vi "Signal Recovery Lockin.vi"(1 "Action":T3=enum."Identify", 2 "Parameters":variant) -> (6 "Output":variant, 7 "Stop":bool)   [LabVIEW 2019]
uses:
  Sub Controls/Instrument Actions.ctl
  Sub Controls/Public.ctl
  Sub Controls/Instrument Match.ctl
  Sub Controls/Scan Output.ctl
  Sub Controls/Instrument IDN.ctl
  Sub Controls/User Event Command.ctl
  <vilib>/Instr/_visa.llb/VISA GPIB Control REN Mode.ctl
panel:
  in  "X/Y":bool=TRUE
  out "Title":string="Signal Recovery Lockin"
  in  "VISA resource name":refnum<visa-resource-name>
  in  "Instruments":T1[](array[typedef])=[{"Model"="7265", "Manufacturer"="Signal Recovery", "Term Character"="", "Wait Time (mS)"=0, "Wait for SRQ"=FALSE, "Type"="Lockin"}]
  out "Model":string
  in  "Address":u16(ring)
  in  "Channel":bool
  in  "Public":T2
  out "Measurement":dbl[](array[numeric]) format="%^.3e"
  # "Ch. 1&2"
  # "Ch. 1"
  # "Mag/Phase"
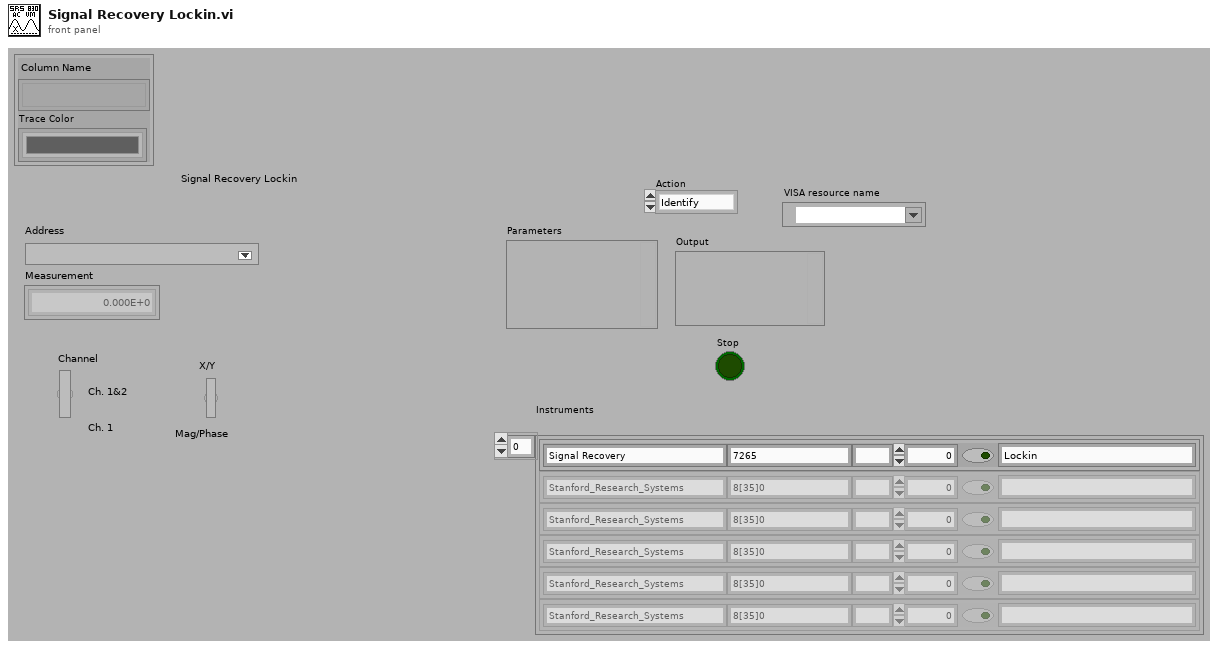
[diagram p1: front panel]
types:
  T1 = typedef "Instrument Match.ctl" = cluster{"Model":string, "Manufacturer":string, "Term Character":string, "Wait Time (mS)":u32, "Wait for SRQ":bool, "Type":string}
  T2 = typedef "Public.ctl" = cluster{"Column Name":string[], "Trace Color":u32[]}
  T3 = typedef "Instrument Actions.ctl" = enum16{"Scan", "Identify", "New", "Configure", "Initialize", "Test", "Read", "Close"}
  T4 = typedef "Scan Output.ctl" = cluster{"Manufacturer":string, "Model":string, "Info":string, "Revision":string, "error out":errorcluster}
  T5 = typedef "Instrument IDN.ctl" = cluster{"VISA Address":string, "Status":u16, "Manufacturer":string, "Model":string, "Info":string, "Info 2":string, "Misc Data":variant}
  T6 = typedef "User Event Command.ctl" = enum32{"Stop Config"}
  T7 = cluster{"VISA resource name":refnum<visa-resource-name>, string}
  T8 = typedef "VISA GPIB Control REN Mode.ctl" = u16
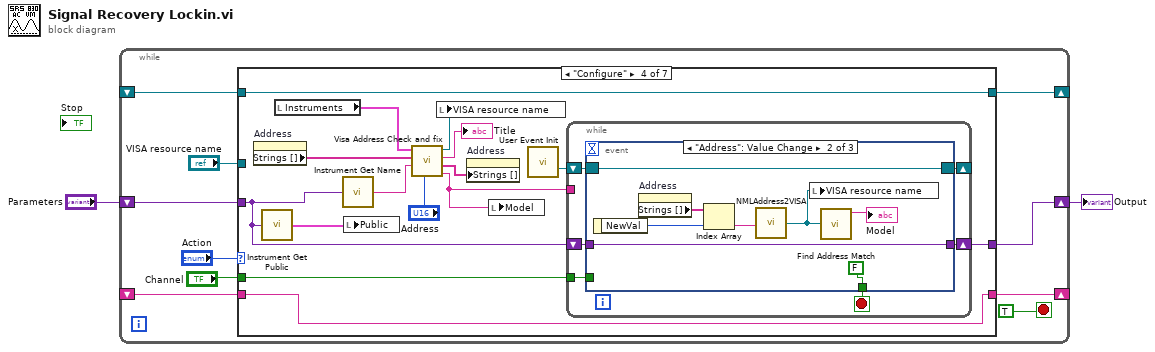
[diagram p0: block diagram]
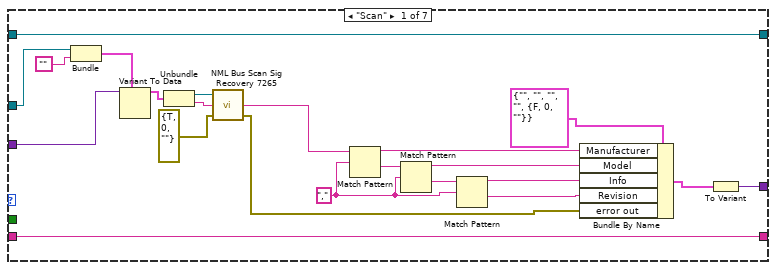
[diagram p2: hidden frame]
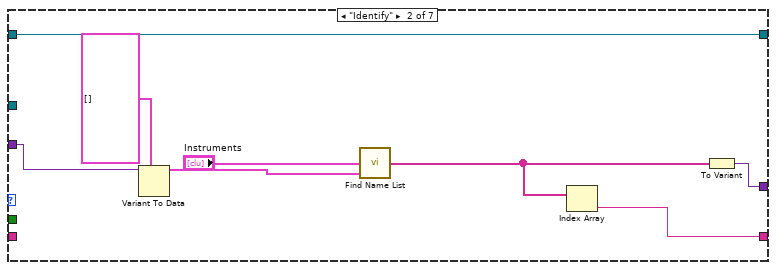
[diagram p3: hidden frame]
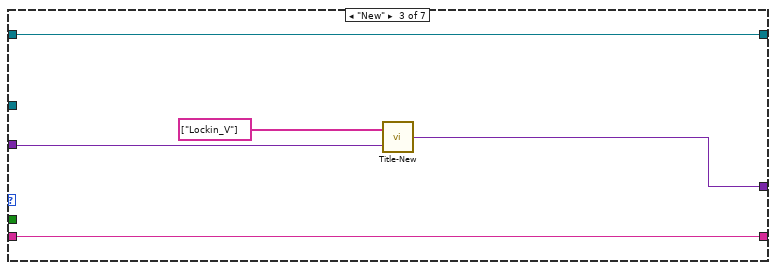
[diagram p4: hidden frame]
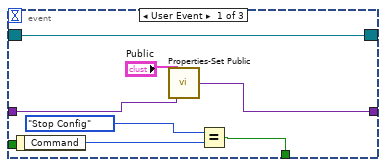
[diagram p5: hidden frame]
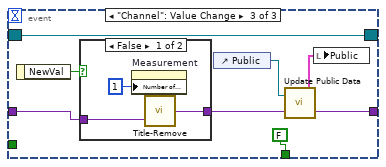
[diagram p6: hidden frame]
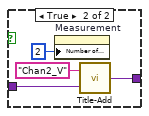
[diagram p7: hidden frame]
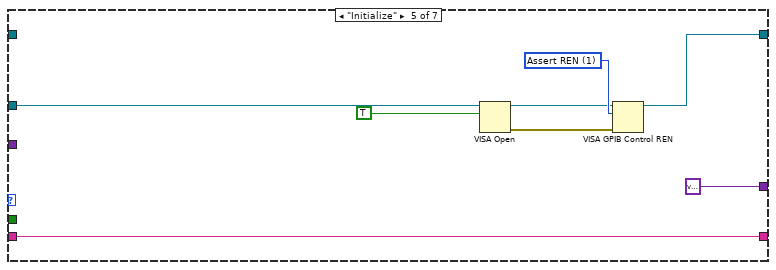
[diagram p8: hidden frame]
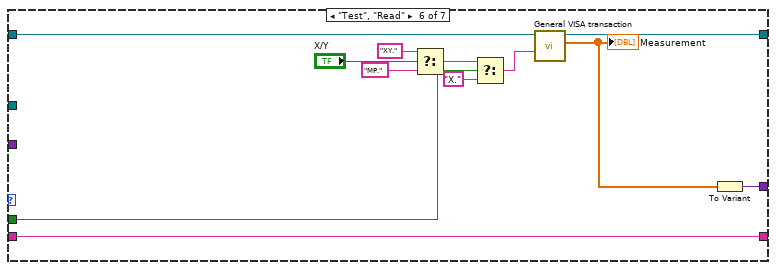
[diagram p9: hidden frame]
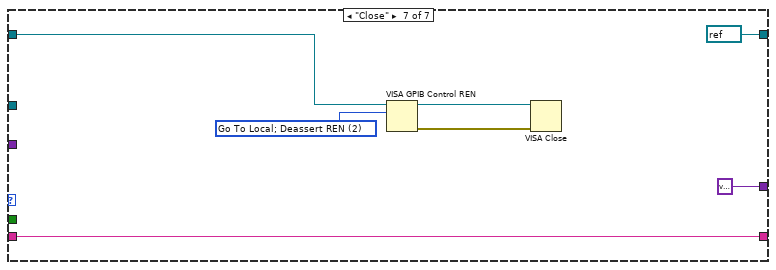
[diagram p10: hidden frame]
diagram:
  n1 = while {
    shift-right: [w11] -> _
    shift-left: _ -> [w10]
    shift-right: [w8] -> w1
    shift-left: "Parameters" -> [w9]
    shift-right: [w4] -> _
    shift-left: _ -> [w3]
    stop <- TRUE stop-if-true
    n2 = case shown="\"Configure\"" "Action" {
      tunnel: [w34 w42 w46 w62 w101 w117 refnum<visa-resource-name> refnum ("Open VISA Resource name")] -> w11
      tunnel: w10 -> [w34 w42 w46 w62 _ w116 w120]
      tunnel: w9 -> [w29 w39 w47 w50 _ _ _]
      tunnel: [w33 w41 w44 w61 variant ("Variant") w118 variant ("Variant")] -> w8
      tunnel: "Channel" -> [_ _ _ w58 _ w108 _]
      tunnel: "VISA resource name" -> [w28 _ _ _ w100 _ _]
      tunnel: [w32 w35 w43 w57 w99 w114 w119] -> w4
      tunnel: w3 -> [w32 _ w43 w57 w99 w114 w119]
      frame "Scan" {
        w21 = ","
        n3 = Bundle("VISA resource name"=w28, "") -> (w30:T7)  [unwired: 1 in]
        n4 = Variant To Data(type=w30, Variant=w29) -> (data=w27:T7)  [unwired: 1 in, 1 out]
        n5 = Unbundle(w27) -> ("VISA resource name"=w25:refnum<visa-resource-name>, w24:string)
        n6 = call "NML Bus Scan Sig Recovery 7265.vi"("error in (no error)"=errorcluster {"status"=TRUE, "code"=0, "source"=""} ("error out"), "String Read In"=w24, "VISA Session"=w25) -> ("error out"=w13:errorcluster, "String Read Out"=w14:string)  [unwired: 1 out]
        n7 = Match Pattern(string=w14, regular expression=w21) -> (before substring=w16:string, after substring=w23:string)  [unwired: 1 in, 2 out]
        n8 = Match Pattern(string=w23, regular expression=w21) -> (before substring=w17:string, after substring=w22:string)  [unwired: 1 in, 2 out]
        n9 = Match Pattern(string=w22, regular expression=w21) -> (before substring=w18:string, after substring=w19:string)  [unwired: 1 in, 2 out]
        n10 = Bundle By Name(cluster=T4 {"Manufacturer"="", "Model"="", "Info"="", "Revision"="", "error out"={"status"=FALSE, "code"=0, "source"=""}} ("Scan Output"), "Manufacturer"=w16, "Model"=w17, "Info"=w18, "Revision"=w19, "error out"=w13) -> (w15:T4)
        n11 = To Variant(anything=w15) -> (Variant=w33:variant)
      }
      frame "Identify" {
        n12 = Variant To Data(type=T5[] [], Variant=w39) -> (data=w37:T5[])  [unwired: 1 in, 1 out]
        n13 = call "Find Name List.vi"("Bus Scan"=w37, "Instruments"="Instruments") -> ("Names"=w36:string[])  [unwired: 1 in]
        n14 = Index Array(array=w36) -> (element=w35:string)  [unwired: 1 in]
        n15 = To Variant(anything=w36) -> (Variant=w41:variant)
      }
      frame "New" {
        n16 = call "Title-New.vi"("Parameters"=w47, "Array"=string[] ["Lockin_V"]) -> ("Instrument Prop"=w44:variant)
      }
      frame "Configure" {
        n17 = property on="Address" class="Ring (strict)"() -> ("Strings []"=w55:string[])  [unwired: 2 in, 2 out]
        n18 = call "Instrument Get Public.vi"("Variant"=w50) -> ("Public"=w60:T2)
        n19 = local read "Instruments"() -> (w49:T1[])
        n20 = call "Instrument Get Name.vi"("Parameters"=w50) -> ("Type"=w51:string)
        n21 = local write "Public"(w60) -> ()
        n22 = call "Visa Address Check and fix.vi"("Address"="Address", "Name"=w51, "NML Addresses"=w55, "Instruments"=w49) -> ("Model"=w52:string, "NML Addresses"=w53:string[], "Title"=→"Title":string, "VISA resource name"=w54:refnum<visa-resource-name>)  [unwired: 2 out]
        n23 = local write "VISA resource name"(w54) -> ()
        n24 = property on="Address" class="Ring (strict)"("Strings []"=w53) -> ()  [unwired: 2 in, 2 out]
        n25 = local write "Model"(w52) -> ()
        n26 = call "User Event Init.vi"() -> ("Event Registration Refnum"=w59:refnum<event-registration>)  [unwired: 14 in, 1 out]
        n27 = while {
          shift-right: [w68] -> w61
          shift-left: w50 -> [w67]
          shift-right: [w64] -> _
          shift-left: w59 -> [w65]
          tunnel: w58 -> [w63]
          tunnel: w52 -> [_]
          stop <- w66 stop-if-true
          n28 = event shown="[1] \"Address\": Value Change" {
            selector: w65 -> [w69 w83 w89]
            dyn-events: [w69 w83 w89] -> w64
            timeout: _ -> [_ _ _]
            tunnel: [w71 FALSE FALSE] -> w66
            tunnel: w67 -> [w74 w77 w90]
            tunnel: [w75 w77 w87] -> w68
            tunnel: w63 -> [_ _ _]
            event User Event {
              n29 = event-data() -> ("Command"=w73:T6)  [unwired: 1 in]
              n30 = call "Properties-Set Public.vi"("Variant"=w74, "New Public"="Public") -> ("Variant 2"=w75:variant)
              n31 = Equal?(x=User_Event_Command."Stop Config", y=w73) -> (x = y?=w71:bool)
            }
            event "Address": Value Change {
              n32 = event-data() -> ("NewVal"=w81:u16)  [unwired: 1 in]
              n33 = property on="Address" class="Ring (strict)"() -> ("Strings []"=w80:string[])  [unwired: 2 in, 2 out]
              n34 = Index Array(array=w80, index=w81) -> (element=w79:string)
              n35 = call "NMLAddress2VISA.vi"("NML Address"=w79) -> ("VISA resource name"=w76:refnum<visa-resource-name>)
              n36 = local write "VISA resource name"(w76) -> ()
              n37 = call "Find Address Match.vi"("VISA resource name"=w76) -> ("Model"=→"Model":string)  [unwired: 3 in, 3 out]
            }
            event "Channel": Value Change {
              n38 = event-data() -> ("NewVal"=w91:bool)  [unwired: 1 in]
              n39 = case shown="False" w91 {
                tunnel: w90 -> [w94 w98]
                tunnel: [w93 w97] -> w88
                frame False {
                  n40 = property on="Measurement" class="Arr (strict)"("Number of Columns"=u32 1) -> ()  [unwired: 2 in, 2 out]
                  n41 = call "Title-Remove.vi"("Parameters"=w94) -> ("Variant"=w93:variant)  [unwired: 1 in]
                }
                frame True {
                  n42 = property on="Measurement" class="Arr (strict)"("Number of Columns"=u32 2) -> ()  [unwired: 2 in, 2 out]
                  n43 = call "Title-Add.vi"("Parameters"=w98, "String"="Chan2_V") -> ("Variant"=w97:variant)
                }
              }
              n44 = control-ref of="Public"() -> (w85:refnum<vi>)
              n45 = call "Update Public Data.vi"("Variant In"=w88, "Public 2"=w85) -> ("Variant Out"=w87:variant, "Public"=w86:T2)
              n46 = local write "Public"(w86) -> ()
            }
          }
        }
      }
      frame "Initialize" {
        w105 = T8 1 items=["Deassert REN", "Assert REN", "Go To Local; Deassert REN ", "Assert REN; Address Device", "Local Lockout (Addressed Devices)", "Local Lockout (This Device)", "Go To Local"] ("Mode")
        n47 = VISA Open(duplicate session (F)=TRUE, VISA resource name=w100) -> (VISA resource name=w103:refnum<visa-resource-name>, error out=w104:errorcluster)  [unwired: 3 in]
        n48 = VISA GPIB Control REN(8:w104, 10:w105, 11:w103) -> (3:w101:refnum<visa-resource-name>)  [unwired: 1 out]
      }
      frame "Test", "Read" {
        n49 = Select(t="XY.", s="X/Y", f="MP.") -> (s? t:f=w111:string)
        n50 = Select(t=w111, s=w108, f="X.") -> (s? t:f=w109:string)
        n51 = call "General VISA transaction.vi"("Command String"=w109, "VISA Session"=w116) -> ("Measurement"=w115:dbl[], "dup VISA Session"=w117:refnum<visa-resource-name>)  [unwired: 4 in, 4 out]
        "Measurement" <- w115
        n52 = To Variant(anything=w115) -> (Variant=w118:variant)
      }
      frame "Close" {
        w124 = T8 2 items=["Deassert REN", "Assert REN", "Go To Local; Deassert REN ", "Assert REN; Address Device", "Local Lockout (Addressed Devices)", "Local Lockout (This Device)", "Go To Local"] ("Mode")
        n53 = VISA GPIB Control REN(10:w124, 11:w120) -> (0:w123:errorcluster, 3:w122:refnum<visa-resource-name>)  [unwired: 1 in]
        n54 = VISA Close(VISA resource name=w122, error in (no error)=w123) -> ()  [unwired: 1 out]
      }
    }
  }
  "Output" <- w1
